vi "PictToU8.lv7.vi"(7 "picture":picture, 11 "Draw Area Size":cluster{"Width":u32, "Height":u32}) -> (4 "image size":i32=34026, 6 "image rect":T2={"left"=0, "top"=0, "right"=107, "bottom"=106}, 8 "image depth":i32=24, 10 "24bit image [U8]":u8[](array[numeric]), 13 "image data":T1, 15 "Draw Area Size out":cluster{"Width":u32, "Height":u32})   [LabVIEW 2024]
panel:
  out "picture":refnum<vi>
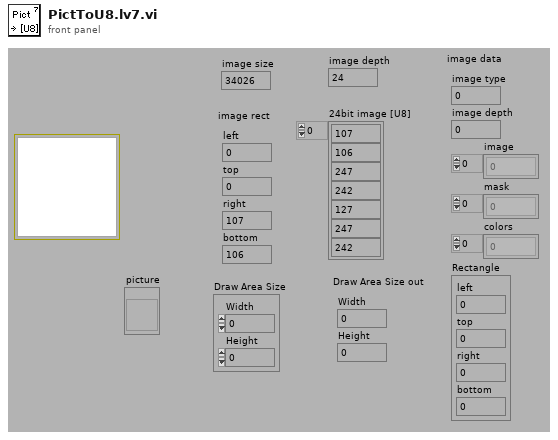
[diagram p1: front panel]
types:
  T1 = cluster{"image type":i32, "image depth":i32, "image":u8[], "mask":u8[], "colors":u32[], "Rectangle":cluster{"left":i16, "top":i16, "right":i16, "bottom":i16}}
  T2 = cluster{"left":i16, "top":i16, "right":i16, "bottom":i16}
  T3 = typedef "imagedata.ctl" = cluster{"image type":i32, "image depth":i32, "image":u8[], "mask":u8[], "colors":u32[], "Rectangle":cluster{"left":i16, "top":i16, "right":i16, "bottom":i16}}
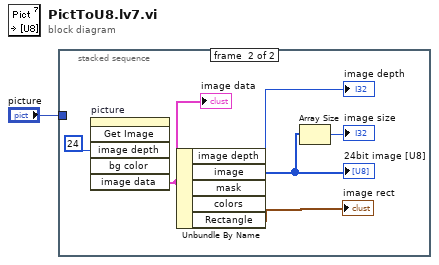
[diagram p0: block diagram]
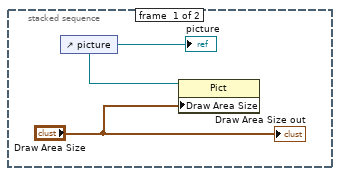
[diagram p2: hidden frame]
diagram:
  n1 = stacked-sequence {
    tunnel: "picture" -> [_ _]
    frame #0 {
      n2 = control-ref of="picture"() -> (w3:refnum<vi>)
      "picture" <- w3
      n3 = property class="Pict"(reference=w3, "Draw Area Size"="Draw Area Size") -> ()  [unwired: 1 in, 2 out]
      "Draw Area Size out" <- "Draw Area Size"
    }
    frame #1 {
      n4 = invoke on="picture" class="Pict" method="Get Image"("image depth"=24) -> ("image data"=w7:T3)  [unwired: 5 in, 5 out]
      "image data" <- w7
      n5 = Unbundle By Name(w7) -> ("image depth"=→"image depth":i32, "image"=w4:u8[], "Rectangle"=→"image rect":T2)  [unwired: 2 out]
      "24bit image [U8]" <- w4
      n6 = Array Size(array=w4) -> (size(s)=→"image size":i32)
    }
  }
